vi "main.vi"() -> ()   [LabVIEW 2025]
uses:
  <userlib>/Nanonis Prog Interface V5/Nanonis Prog Interface.lvlib
panel:
  out "FRC":sgl format="%#_3g"
  out "CCR":sgl
  in  "Ref_filepath":path=path "si111-cornerhole.npy" caption="filename"
  in  "Final Overvew Details":T1={"Size (m)"={"Width"=nan, "Height"=nan}, "Pixels"=0, "Scan Speed (m/s)"=nan}
  in  "Shaping Attempt 5":T2={"Tip Lift (m)"=-1.3e-09, "Lifting Bias (V)"=5.0, "# Iterations"=20} caption="Tip Lift 1" {"# Iterations" step=1; "Lifting Bias (V)" step=0.5 format="%#_5g"; "Tip Lift (m)" step=5e-11 format="%.2p"}
  in  "Shaping Attempt 4":T2={"Tip Lift (m)"=-1.3e-09, "Lifting Bias (V)"=5.0, "# Iterations"=20} caption="Tip Lift 1" {"# Iterations" step=1; "Lifting Bias (V)" step=0.5 format="%#_5g"; "Tip Lift (m)" step=5e-11 format="%.2p"}
  in  "Shaping Attempt 3":T2={"Tip Lift (m)"=-1.3e-09, "Lifting Bias (V)"=5.0, "# Iterations"=20} caption="Tip Lift 1" {"# Iterations" step=1; "Lifting Bias (V)" step=0.5 format="%#_5g"; "Tip Lift (m)" step=5e-11 format="%.2p"}
  in  "Shaping Attempt 2":T2={"Tip Lift (m)"=-1.3e-09, "Lifting Bias (V)"=5.0, "# Iterations"=20} caption="Tip Lift 1" {"# Iterations" step=1; "Lifting Bias (V)" step=0.5 format="%#_5g"; "Tip Lift (m)" step=5e-11 format="%.2p"}
  in  "Tip Shaping Position":cluster{"X (m)":sgl, "Y (m)":sgl} {"X (m)" format="%#_6p"; "Y (m)" format="%#_6p"}
  out "Vy vs. Scan #":picture
  out "Vx vs. Scan #":picture
  out "Next filename":path caption="filename"
  in  "Ref Info":cluster{"Scan Size (m)":sgl, "Pixels":i32}={"Scan Size (m)"=2e-08, "Pixels"=720} {"Scan Size (m)" format="%#_4p"}
  out "Time \nElapsed (s)":dbl format="%#.2f"
  out "Shaping\nAttempts":i32
  in  "Shaping Attempt 1":T2={"Tip Lift (m)"=-1.3e-09, "Lifting Bias (V)"=5.0, "# Iterations"=20} caption="Tip Lift 1" {"# Iterations" step=1; "Lifting Bias (V)" step=0.5 format="%#_5g"; "Tip Lift (m)" step=5e-11 format="%.2p"}
  out "Finished?":bool
  in  "Start":bool
  # "Auto Tip Shaper"
  # "Tip Shaping Controls"
  # "Drift Plots"
  # "Pre-checks"
  # "See readme at https://github.com/DS-Barker/stm-tip-classifier for instructions"
  # "Final Overview Settings"
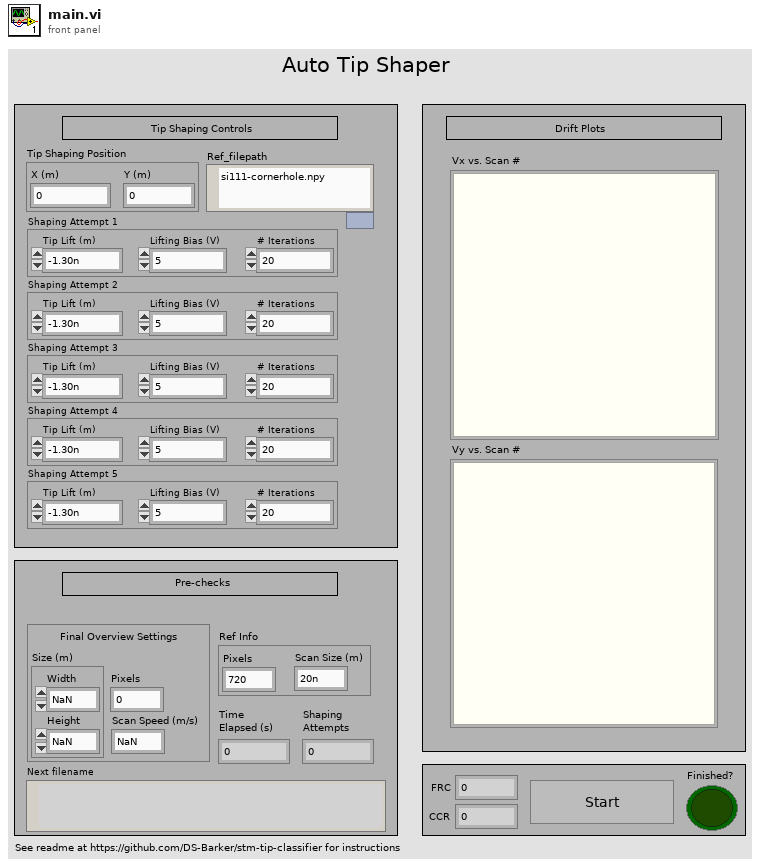
[diagram p1: front panel]
types:
  T1 = cluster{"Size (m)":cluster{"Width":sgl, "Height":sgl}, "Pixels":i32, "Scan Speed (m/s)":sgl}
  T2 = cluster{"Tip Lift (m)":dbl, "Lifting Bias (V)":dbl, "# Iterations":i32}
  T3 = cluster{cluster{"x":sgl, "y":sgl}[], cluster{"x":sgl, "y":sgl}[], cluster{"x":sgl, "y":sgl}[]}
  T4 = enum16{"Init", "Scanning", "Resolve Tip", "Shaping 1", "Shaping 2", "Shaping 3", "Shaping 4", "Shaping 5", "Move Away", "Quit"}
  T5 = cluster{"Application ref out":refnum<vi>, "error out":errorcluster, "Corner Coords":cluster{"Corner x":sgl, "Corner y":sgl}, "Tip Shaping Position":cluster{"Tip x (m)":sgl, "Tip y (m)":sgl}, "Session path":path, "Filenames":cluster{"Filename 1":path, "Filename 2":path}, "Downscale Info":cluster{"Scale factor":sgl, "Downscale ref/input":string}}
  T6 = cluster{"Scale factor":sgl, "Downscale ref/input":string}
  T7 = cluster{"Tip Lift 1 (m)":dbl, "Lift Time 1 (s)":dbl}
  T8 = cluster{"Bias Lift (V)":dbl, "Bias Settling Time (s)":dbl}
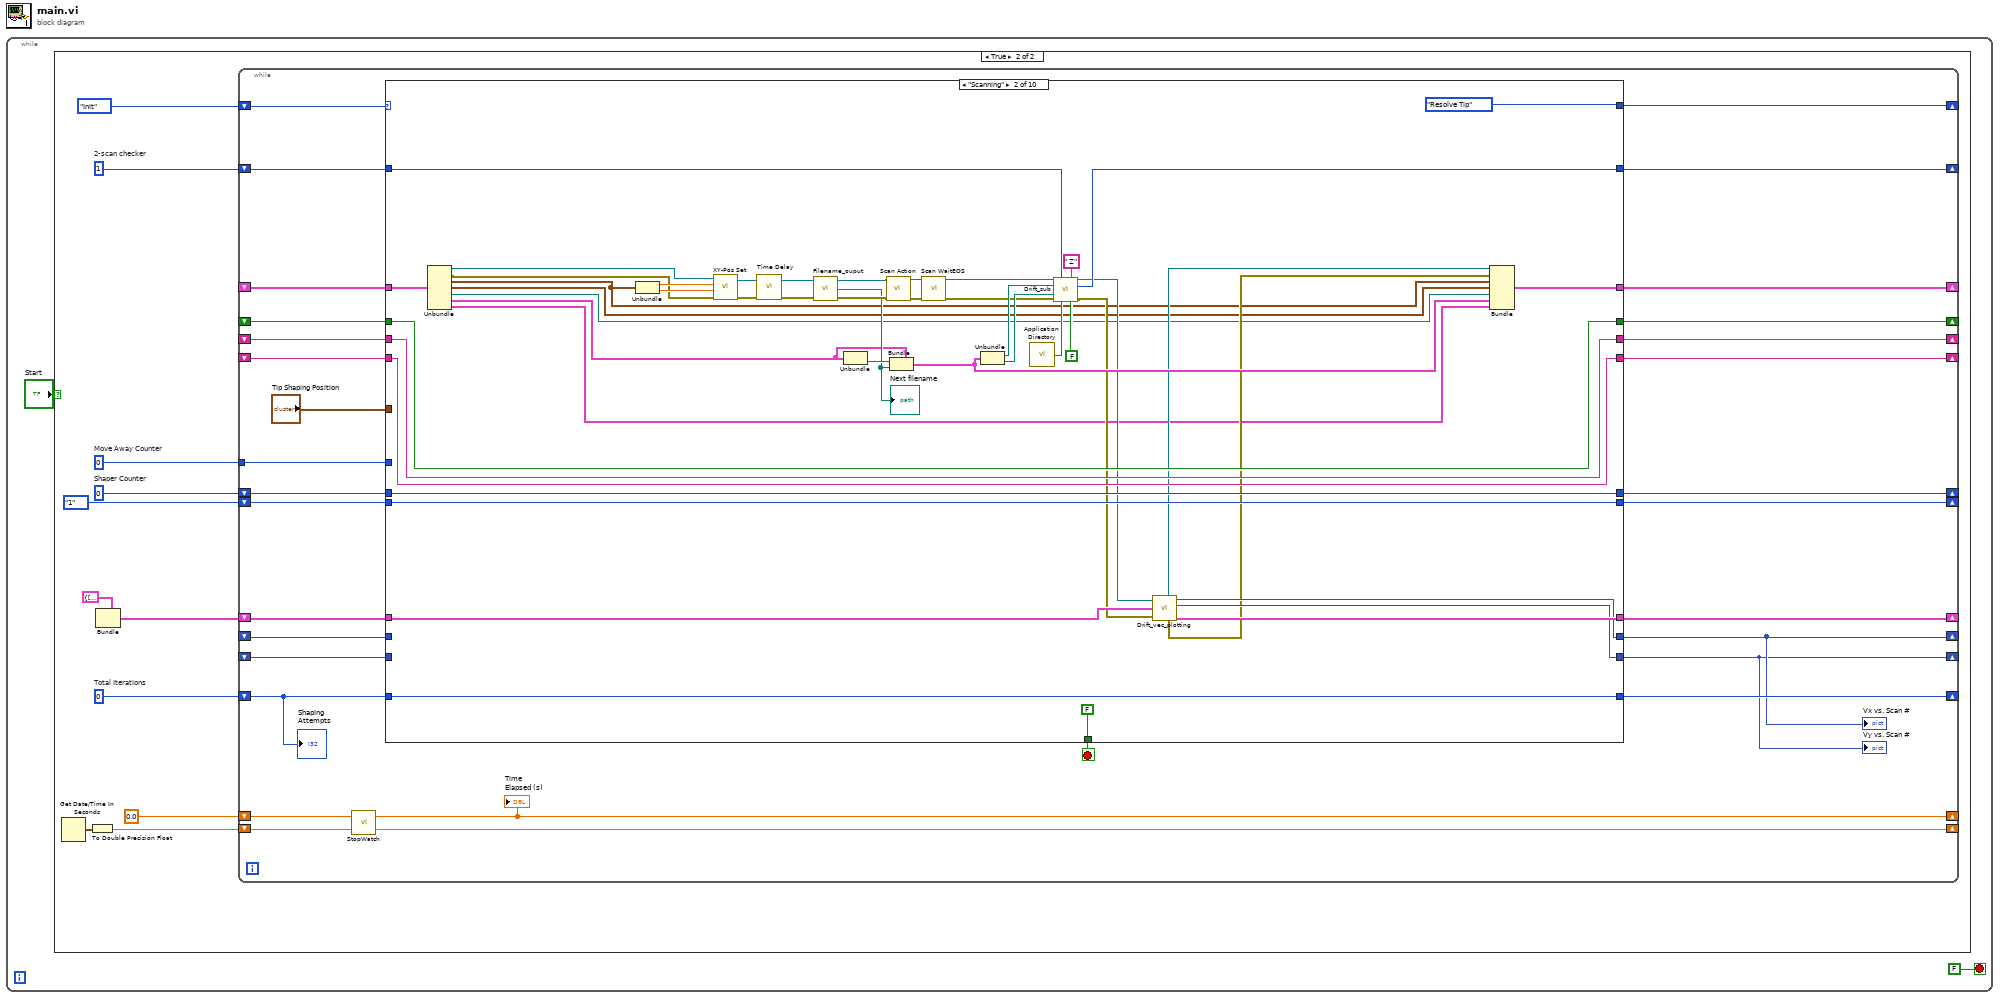
[diagram p0: block diagram]
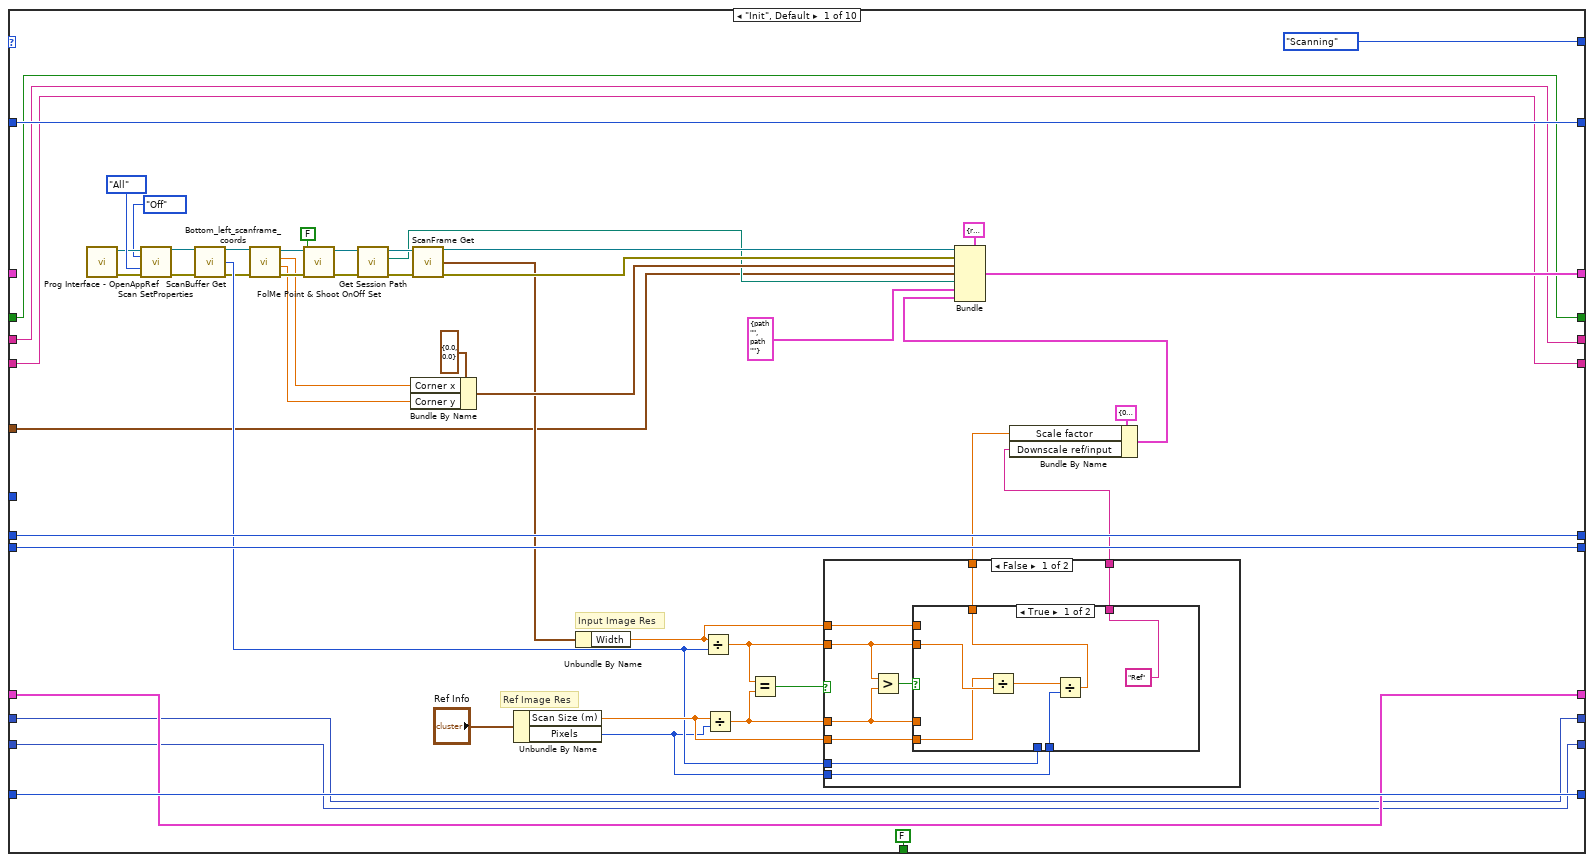
[diagram p3: hidden frame]
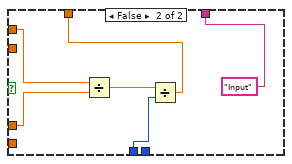
[diagram p4: hidden frame]
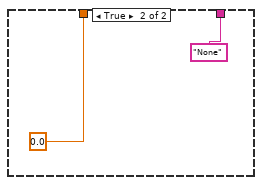
[diagram p5: hidden frame]
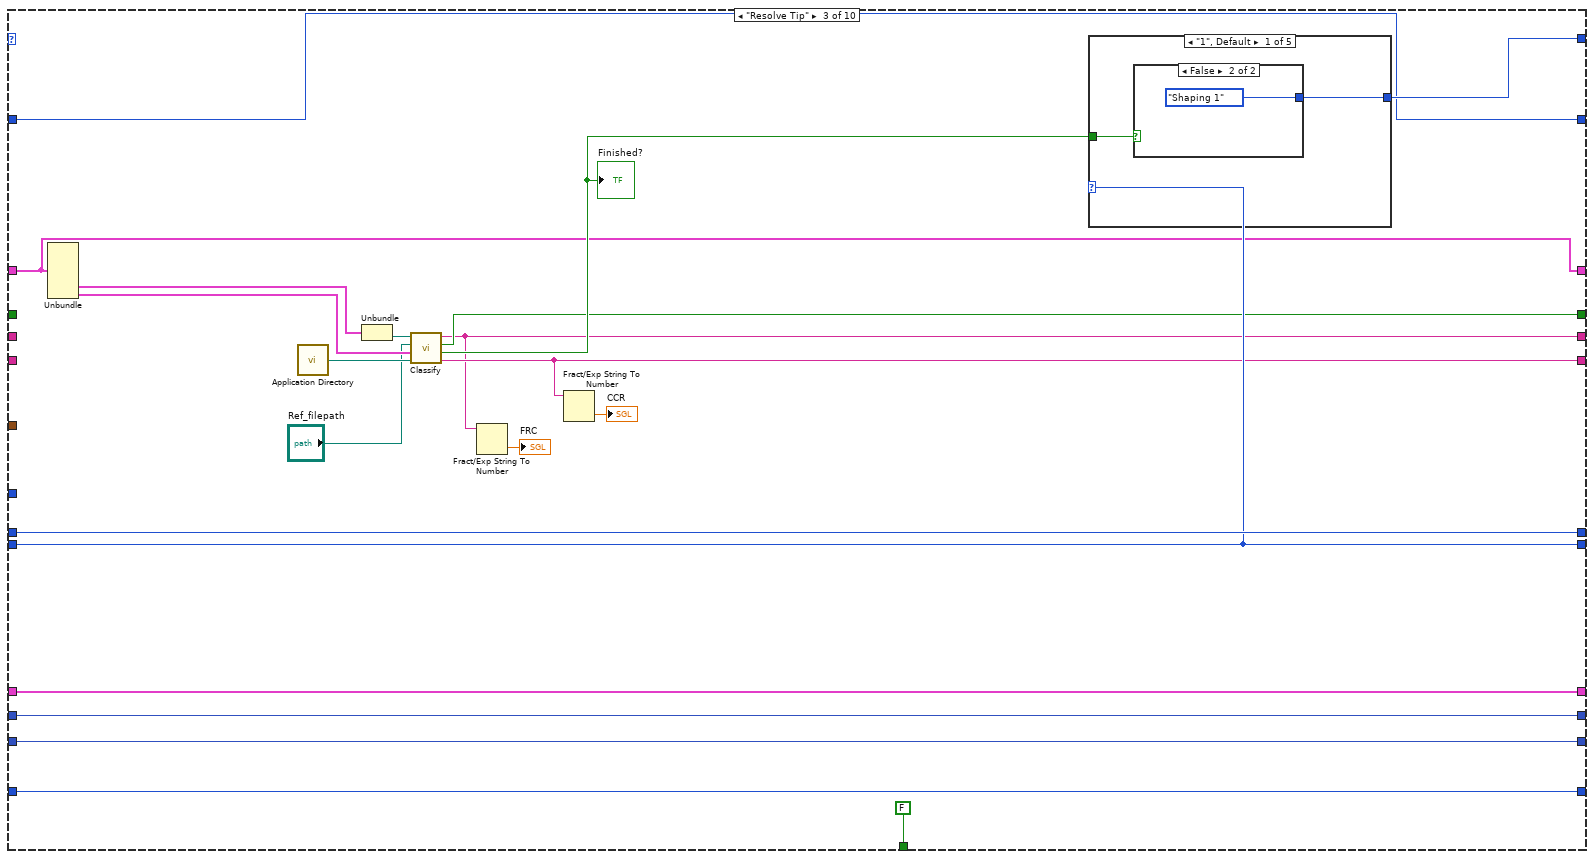
[diagram p6: hidden frame]
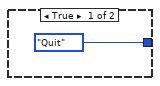
[diagram p7: hidden frame]
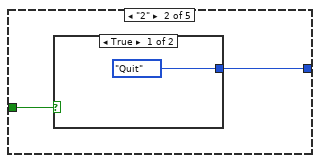
[diagram p8: hidden frame]
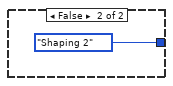
[diagram p9: hidden frame]
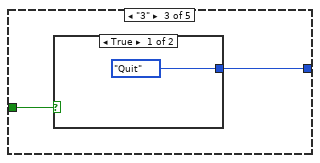
[diagram p10: hidden frame]
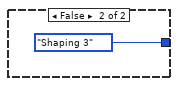
[diagram p11: hidden frame]
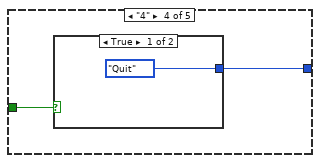
[diagram p12: hidden frame]
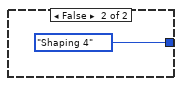
[diagram p13: hidden frame]
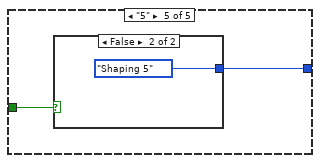
[diagram p14: hidden frame]
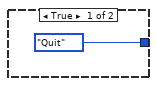
[diagram p15: hidden frame]
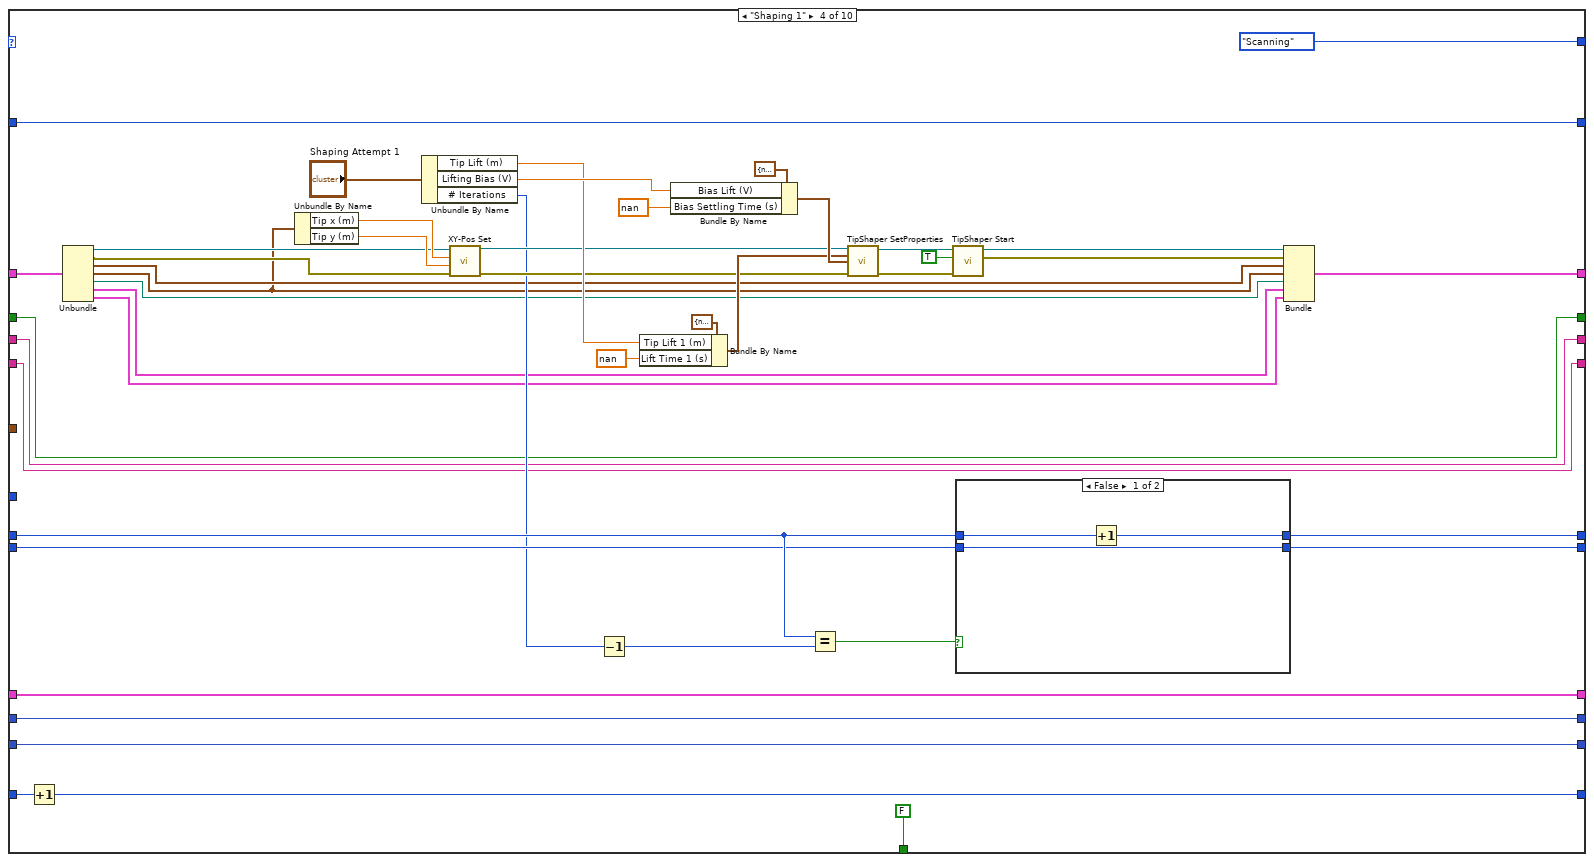
[diagram p16: hidden frame]
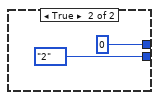
[diagram p17: hidden frame]
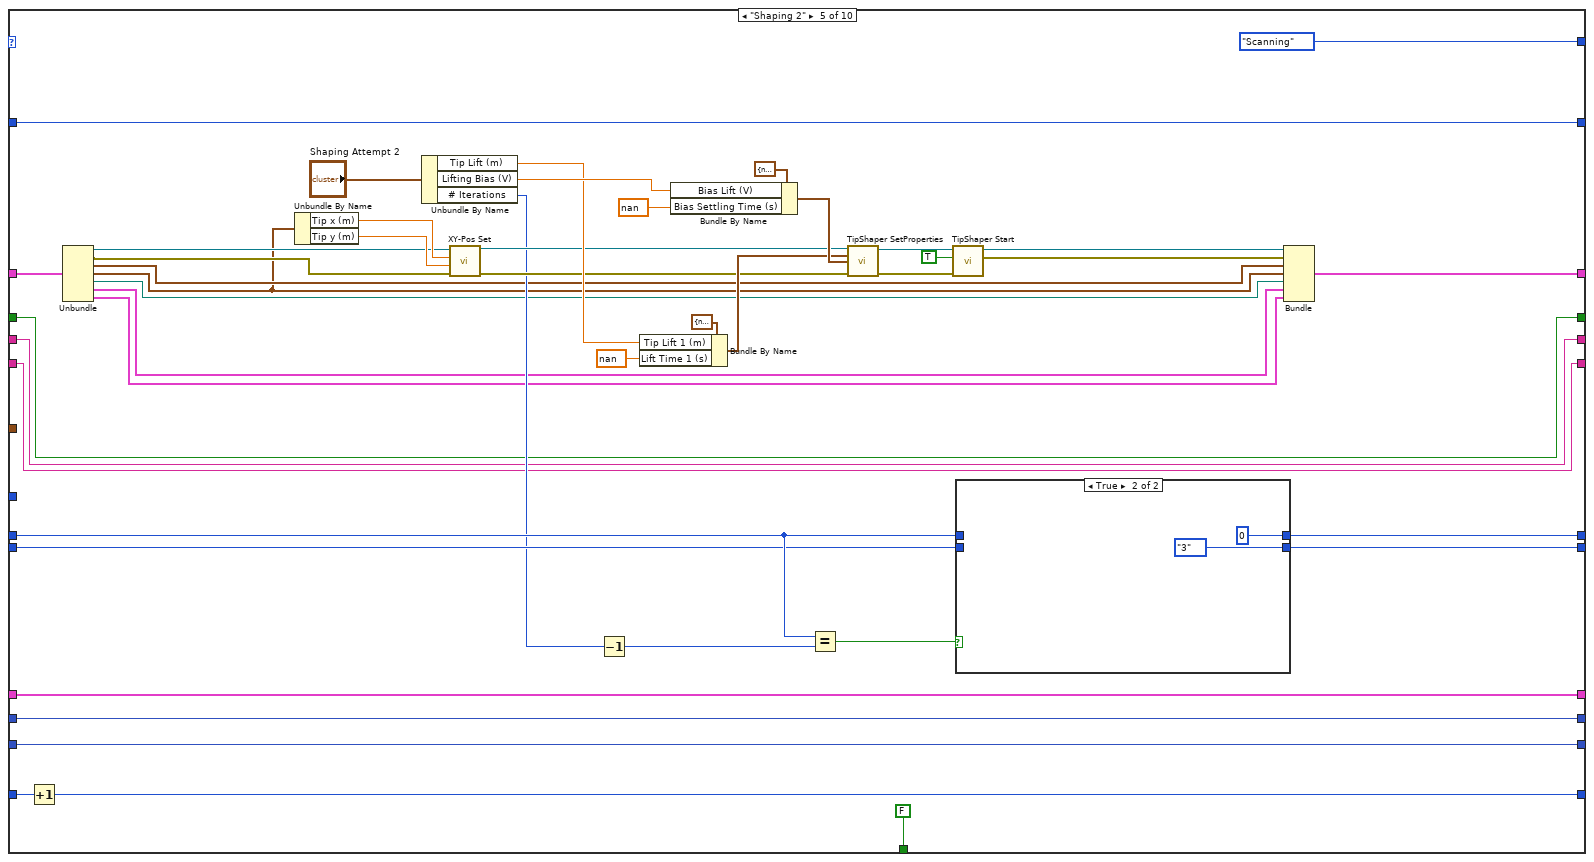
[diagram p18: hidden frame]
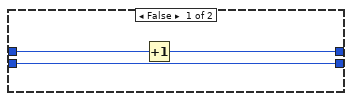
[diagram p19: hidden frame]
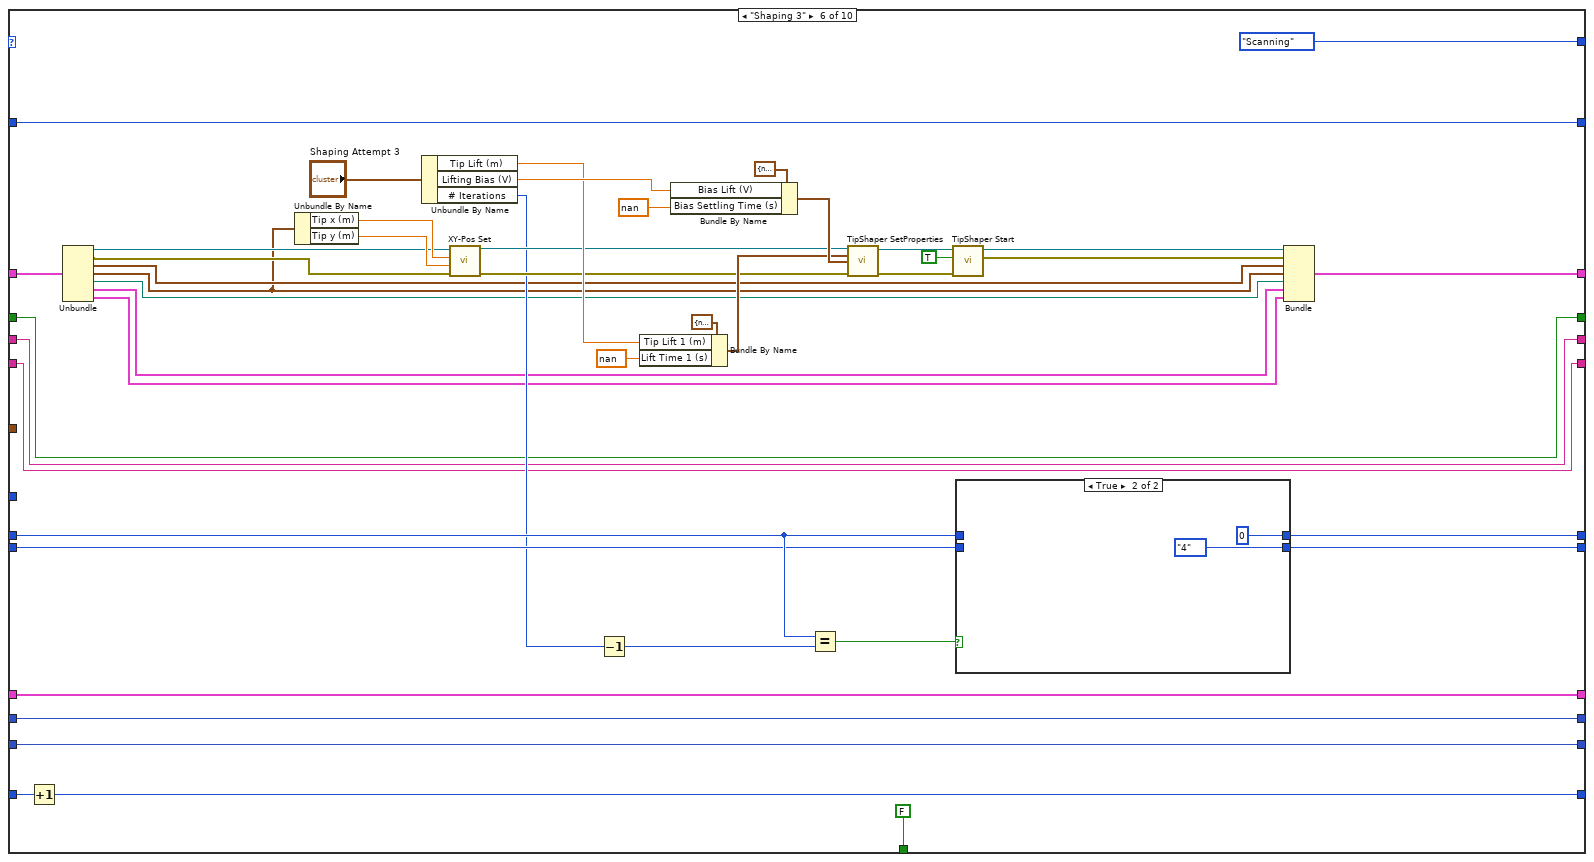
[diagram p20: hidden frame]
diagram:
  n1 = while {
    stop <- FALSE stop-if-true
    n2 = case shown="True" "Start" {
      frame False {
      }
      frame True {
        w5 = 1  # 2-scan checker
        w9 = 0  # Total Iterations
        w10 = 0  # Move Away Counter
        w12 = 0  # Shaper Counter
        n3 = Get Date/Time In Seconds() -> (seconds since 1Jan1904=w8:timestamp)
        n4 = To Double Precision Float(number=w8) -> (double precision float=w7:dbl)
        n5 = Bundle(cluster=T3 {[], [], []} ("output cluster")) -> (w4:T3)  [unwired: 3 in]
        n6 = while {
          shift-right: [w41] -> _
          shift-left: T4."Init" -> [w44]
          shift-right: [w43] -> _
          shift-left: _ -> [w42]
          shift-right: [w38] -> _
          shift-left: w12 -> [w39]
          shift-right: [w36] -> _
          shift-left: enum16{"1", "2", "3", "4", "5"}."1" -> [w37]
          tunnel: w10 -> [w35]
          shift-right: [w33] -> _
          shift-left: w9 -> [w34]
          shift-right: [w32] -> _
          shift-left: 0.0 ("Elapsed Time (Secs)") -> [w30]
          shift-right: [w31] -> _
          shift-left: w7 -> [w29]
          shift-right: [w27] -> _
          shift-left: w5 -> [w28]
          shift-right: [w25] -> _
          shift-left: w4 -> [w26]
          shift-right: [w24] -> _
          shift-left: _ -> [w22]
          shift-right: [w23] -> _
          shift-left: _ -> [w21]
          shift-right: [w18] -> _
          shift-left: _ -> [w15]
          shift-right: [w19] -> _
          shift-left: _ -> [w16]
          shift-right: [w20] -> _
          shift-left: _ -> [w17]
          stop <- w40 stop-if-true
          n7 = call "StopWatch.vi"("Global In (s)"=w29, "Elapsed In (s)"=w30) -> ("Global Out (s)"=w31:dbl, "Elapsed Time (Secs)"=w32:dbl)  [unwired: 1 in]
          "Time \nElapsed (s)" <- w32
          n8 = case shown="\"Scanning\"" w44 {
            selector: w44 -> [_ _ _ _ _ _ _ _ _ w533]
            tunnel: [w90 w159 w172 w232 w282 w332 w382 w432 w474 w507] -> w43
            tunnel: w42 -> [_ w126 w172 w213 w263 w313 w363 w414 w475 w513]
            tunnel: [T4."Scanning" T4."Resolve Tip" w184 T4."Scanning" T4."Scanning" T4."Scanning" T4."Scanning" w406 w467 w533] -> w41
            tunnel: [FALSE FALSE FALSE FALSE FALSE FALSE FALSE FALSE FALSE TRUE] -> w40
            tunnel: w39 -> [w85 w157 w183 w230 w280 w330 w380 w430 w473 w534]
            tunnel: [w85 w157 w183 w231 w281 w331 w381 w431 w473 w534] -> w38
            tunnel: w37 -> [w84 w156 w182 w226 w276 w326 w376 w427 w472 w531]
            tunnel: [w84 w156 w182 w228 w278 w328 w378 w428 w472 w531] -> w36
            tunnel: w35 -> [_ _ _ _ _ _ _ _ w471 _]
            tunnel: [w82 w154 w181 w221 w271 w321 w371 w422 w465 w532] -> w33
            tunnel: w34 -> [w82 w154 w181 w222 w272 w322 w372 w423 w465 w532]
            tunnel: w28 -> [w63 w146 w180 w220 w270 w320 w370 w421 w464 w530]
            tunnel: [w63 w145 w180 w220 w270 w320 w370 w421 w464 w530] -> w27
            tunnel: [w55 w132 w166 w215 w265 w315 w365 w416 w459 _] -> w19
            tunnel: [w54 w133 w168 w216 w266 w316 w366 w417 w460 _] -> w18
            tunnel: [w56 w131 w176 w214 w264 w314 w364 w415 w458 _] -> w20
            tunnel: [w59 w137 w175 w219 w269 w319 w369 w420 w463 w506] -> w25
            tunnel: [w58 w136 w174 w218 w268 w318 w368 w419 w462 w500] -> w24
            tunnel: [w57 w135 w173 w217 w267 w317 w367 w418 w461 w499] -> w23
            tunnel: w26 -> [w59 w134 w175 w219 w269 w319 w369 w420 w463 w506]
            tunnel: w22 -> [w58 _ w174 w218 w268 w318 w368 w419 w462 w500]
            tunnel: w21 -> [w57 _ w173 w217 w267 w317 w367 w418 w461 w499]
            tunnel: w17 -> [w56 w131 _ w214 w264 w314 w364 w415 w458 _]
            tunnel: w16 -> [w55 w132 _ w215 w265 w315 w365 w416 w459 _]
            tunnel: w15 -> [w54 w133 _ w216 w266 w316 w366 w417 w460 _]
            tunnel: "Tip Shaping Position" -> [w47 _ _ _ _ _ _ _ _ _]
            frame "Init", Default {
              # "Ref Image Res"
              # "Input Image Res"
              n9 = call <userlib>:"Prog Interface - OpenAppRef.vi"() -> ("Error out"=w93:errorcluster, "Application reference"=w94:refnum<vi>)  [unwired: 6 in]
              n10 = call <userlib>:"Scan SetProperties.vi"("Application ref in"=w94, "Continuous scan"=enum16{"No change", "On", "Off"}."Off", "Auto save"=enum16{"No change", "All", "Next", "Off"}."All", "Error in (no error)"=w93) -> ("Application ref out"=w76:refnum<vi>, "Error out"=w75:errorcluster)  [unwired: 10 in]
              n11 = call <userlib>:"ScanBuffer Get.vi"("Application ref in"=w76, "error in (no error)"=w75) -> ("Application ref out"=w53:refnum<vi>, "Pixels/line"=w62:i32, "error out"=w52:errorcluster)  [unwired: 9 in, 2 out]
              n12 = call "Bottom_left_scanframe_coords.vi"("error in"=w52, "Application ref in"=w53) -> ("error out"=w50:errorcluster, "Y_bl"=w48:sgl, "X_bl"=w49:sgl, "Application ref out"=w51:refnum<vi>)  [unwired: 2 in]
              n13 = call <userlib>:"FolMe Point & Shoot OnOff Set.vi"("error in (no error)"=w50, "Point & Shoot On/Off"=FALSE, "Application ref in"=w51) -> ("error out"=w80:errorcluster, "Application ref out"=w81:refnum<vi>)  [unwired: 7 in]
              n14 = call <userlib>:"Get Session Path.vi"("error in (no error)"=w80, "Application ref in"=w81) -> ("error out"=w78:errorcluster, "Session path"=w77:path, "Application ref out"=w79:refnum<vi>)  [unwired: 7 in]
              n15 = Bundle By Name(cluster=cluster{"Corner x":sgl, "Corner y":sgl} {"Corner x"=0.0, "Corner y"=0.0} ("Corner Coords"), "Corner x"=w49, "Corner y"=w48) -> (w87:cluster{"Corner x":sgl, "Corner y":sgl})
              n16 = call <userlib>:"ScanFrame Get.vi"("Application ref in"=w79, "error in (no error)"=w78) -> ("Application ref out"=w92:refnum<vi>, "Size (m)"=w74:cluster{"Width":sgl, "Height":sgl}, "error out"=w91:errorcluster)  [unwired: 9 in, 2 out]
              n17 = Unbundle By Name("Ref Info") -> ("Scan Size (m)"=w69:sgl, "Pixels"=w61:i32)
              n18 = Unbundle By Name(w74) -> ("Width"=w68:sgl)
              n19 = Divide(x=w68, y=w62) -> (x/y=w71:sgl)
              n20 = Divide(x=w69, y=w61) -> (x/y=w70:sgl)
              n21 = Equal?(x=w71, y=w70) -> (x = y?=w72:bool)
              n22 = case shown="False" w72 {
                tunnel: w71 -> [w103 _]
                tunnel: w70 -> [w102 _]
                tunnel: w69 -> [w100 _]
                tunnel: w68 -> [w101 _]
                tunnel: [w99 "None"] -> w66
                tunnel: w62 -> [w98 _]
                tunnel: w61 -> [w97 _]
                tunnel: [w96 sgl 0.0] -> w60
                frame False {
                  n23 = Greater?(x=w103, y=w102) -> (0:w104:bool)
                  n24 = case shown="True" w104 {
                    tunnel: w103 -> [w110 _]
                    tunnel: w102 -> [_ w115]
                    tunnel: w101 -> [_ w116]
                    tunnel: w100 -> [w109 _]
                    tunnel: ["Ref" "Input"] -> w99
                    tunnel: w98 -> [_ w112]
                    tunnel: w97 -> [w106 _]
                    tunnel: [w105 w111] -> w96
                    frame True {
                      n25 = Divide(x=w109, y=w110) -> (x/y=w107:sgl)
                      n26 = Divide(x=w107, y=w106) -> (x/y=w105:sgl)
                    }
                    frame False {
                      n27 = Divide(x=w116, y=w115) -> (x/y=w113:sgl)
                      n28 = Divide(x=w113, y=w112) -> (x/y=w111:sgl)
                    }
                  }
                }
                frame True {
                }
              }
              n29 = Bundle By Name(cluster=T6 {"Scale factor"=0.0, "Downscale ref/input"=""} ("Downscale Info"), "Scale factor"=w60, "Downscale ref/input"=w66) -> (w65:T6)
              n30 = Bundle(cluster=T5 {"Application ref out"=refnum, "error out"={"status"=FALSE, "code"=0, "source"=""}, "Corner Coords"={"Corner x"=0.0, "Corner y"=0.0}, "Tip Shaping Position"={"Tip x (m)"=0.0, "Tip y (m)"=0.0}, "Session path"=path "", "Filenames"={"Filename 1"=path "", "Filename 2"=path ""}, "Downscale Info"={"Scale factor"=0.0, "Downscale ref/input"=""}}, "Application ref out"=w92, "error out"=w91, "Corner Coords"=w87, "Tip Shaping Position"=w47, "Session path"=w77, "Filenames"=cluster{"Filename 1":path, "Filename 2":path} {"Filename 1"=path "", "Filename 2"=path ""}, "Downscale Info"=w65) -> (w90:T5)
            }
            frame "Scanning" {
              n31 = Unbundle(w126) -> ("Application ref out"=w125:refnum<vi>, "error out"=w124:errorcluster, "Corner Coords"=w123:cluster{"Corner x":sgl, "Corner y":sgl}, "Tip Shaping Position"=w122:cluster{"Tip x (m)":sgl, "Tip y (m)":sgl}, "Session path"=w121:path, "Filenames"=w120:cluster{"Filename 1":path, "Filename 2":path}, "Downscale Info"=w119:T6)
              n32 = Unbundle(w123) -> ("Corner x"=w164:sgl, "Corner y"=w163:sgl)
              n33 = call <userlib>:"XY-Pos Set.vi"("error in (no error)"=w124, "Y (m)"=w163, "X (m)"=w164, "Application ref in"=w125) -> ("error out"=w162:errorcluster, "Application ref out"=w151:refnum<vi>)  [unwired: 4 in]
              n34 = call "Time Delay"("error in (no error)"=w162) -> ("error out"=w150:errorcluster)  [unwired: 10 in]
              n35 = call "Filename_ouput.vi"("Error in (no error)"=w150, "Application ref in"=w151) -> ("error out"=w152:errorcluster, "Next filename"=w148:path, "Application ref out"=w153:refnum<vi>)  [unwired: 1 in]
              "Next filename" <- w148
              n36 = Unbundle(w120) -> ("Filename 2"=w149:path)  [unwired: 1 out]
              n37 = call <userlib>:"Scan Action.vi"("error in (no error)"=w152, "Application ref in"=w153) -> ("error out"=w161:errorcluster, "Application ref out"=w160:refnum<vi>)  [unwired: 7 in]
              n38 = Bundle(cluster=w120, "Filename 1"=w149, "Filename 2"=w148) -> (w147:cluster{"Filename 1":path, "Filename 2":path})
              n39 = call <userlib>:"Scan WaitEOS.vi"("error in (no error)"=w161, "Application ref in"=w160) -> ("error out"=w141:errorcluster, "Application ref out"=w144:refnum<vi>)  [unwired: 5 in, 2 out]
              n40 = Unbundle(w147) -> ("Filename 1"=w143:path, "Filename 2"=w142:path)
              n41 = call <vilib>:"Application Directory.vi"() -> ("Application Directory"=w139:path)
              n42 = call "Drift_sub.vi"("Application ref in"=w144, "2-scan checker in"=w146, "Image Channel"=" Z", "Filename_1"=w143, "Filename_2"=w142, "error in"=w141, "Python Directory Path"=w139, "Z-Compensation?"=FALSE) -> ("Application ref out"=w130:refnum<vi>, "2-scan checker out"=w145:i32, "error out"=w128:errorcluster)  [unwired: 5 in]
              n43 = call "Drift_vec_plotting.vi"("Application ref in"=w130, "Plotting Data In"=w134, "error in"=w128) -> ("Application ref out"=w129:refnum<vi>, "Vx vs. Scan #"=w136:picture, "Vy vs. Scan #"=w135:picture, "error out"=w127:errorcluster, "Plotting Data Out"=w137:T3)  [unwired: 2 in, 1 out]
              n44 = Bundle("Application ref out"=w129, "error out"=w127, "Corner Coords"=w123, "Tip Shaping Position"=w122, "Session path"=w121, "Filenames"=w147, "Downscale Info"=w119) -> (w159:T5)  [unwired: 1 in]
            }
            frame "Resolve Tip" {
              n45 = Unbundle(w172) -> ("Filenames"=w171:cluster{"Filename 1":path, "Filename 2":path}, "Downscale Info"=w170:T6)  [unwired: 5 out]
              n46 = call <vilib>:"Application Directory.vi"() -> ("Application Directory"=w179:path)
              n47 = Unbundle(w171) -> ("Filename 2"=w177:path)  [unwired: 1 out]
              n48 = call "Classify.vi"("Python Directory Path"=w179, "input cluster"=w170, "Ref_filepath"="Ref_filepath", "Filename_1"=w177) -> ("CCR"=w168:string, "Good Image"=w178:bool, "Tip Change?"=w176:bool, "FRC"=w166:string)
              "Finished?" <- w178
              n49 = Fract/Exp String To Number(string=w166) -> (number=→"FRC":dbl)  [unwired: 3 in, 1 out]
              n50 = Fract/Exp String To Number(string=w168) -> (number=→"CCR":dbl)  [unwired: 3 in, 1 out]
              n51 = case shown="\"1\", Default" w182 {
                tunnel: w178 -> [w187 w191 w195 w199 w203]
                tunnel: [w186 w190 w194 w198 w202] -> w184
                frame "1", Default {
                  n52 = case shown="False" w187 {
                    tunnel: [T4."Quit" T4."Shaping 1"] -> w186
                    frame True {
                    }
                    frame False {
                    }
                  }
                }
                frame "2" {
                  n53 = case shown="True" w191 {
                    tunnel: [T4."Quit" T4."Shaping 2"] -> w190
                    frame True {
                    }
                    frame False {
                    }
                  }
                }
                frame "3" {
                  n54 = case shown="True" w195 {
                    tunnel: [T4."Quit" T4."Shaping 3"] -> w194
                    frame True {
                    }
                    frame False {
                    }
                  }
                }
                frame "4" {
                  n55 = case shown="True" w199 {
                    tunnel: [T4."Quit" T4."Shaping 4"] -> w198
                    frame True {
                    }
                    frame False {
                    }
                  }
                }
                frame "5" {
                  n56 = case shown="False" w203 {
                    tunnel: [T4."Quit" T4."Shaping 5"] -> w202
                    frame True {
                    }
                    frame False {
                    }
                  }
                }
              }
            }
            frame "Shaping 1" {
              n57 = Increment(x=w222) -> (x+1=w221:i32)
              n58 = Unbundle(w213) -> ("Application ref out"=w212:refnum<vi>, "error out"=w211:errorcluster, "Corner Coords"=w210:cluster{"Corner x":sgl, "Corner y":sgl}, "Tip Shaping Position"=w209:cluster{"Tip x (m)":sgl, "Tip y (m)":sgl}, "Session path"=w208:path, "Filenames"=w207:cluster{"Filename 1":path, "Filename 2":path}, "Downscale Info"=w206:T6)
              n59 = Unbundle By Name(w209) -> ("Tip x (m)"=w238:sgl, "Tip y (m)"=w237:sgl)
              n60 = Unbundle By Name("Shaping Attempt 1") -> ("Tip Lift (m)"=w244:dbl, "Lifting Bias (V)"=w247:dbl, "# Iterations"=w223:i32)
              n61 = call <userlib>:"XY-Pos Set.vi"("error in (no error)"=w211, "Y (m)"=w237, "X (m)"=w238, "Application ref in"=w212) -> ("error out"=w235:errorcluster, "Application ref out"=w236:refnum<vi>)  [unwired: 4 in]
              n62 = Decrement(x=w223) -> (x-1=w224:i32)
              n63 = Bundle By Name(cluster=T7 {"Tip Lift 1 (m)"=nan, "Lift Time 1 (s)"=nan} ("Tip Lift 1"), "Tip Lift 1 (m)"=w244, "Lift Time 1 (s)"=nan) -> (w242:T7)
              n64 = Bundle By Name(cluster=T8 {"Bias Lift (V)"=nan, "Bias Settling Time (s)"=nan} ("Bias Lift"), "Bias Lift (V)"=w247, "Bias Settling Time (s)"=nan) -> (w246:T8)
              n65 = Equal?(x=w230, y=w224) -> (x = y?=w229:bool)
              n66 = call <userlib>:"TipShaper SetProperties.vi"("Application ref in"=w236, "Tip Lift 1"=w242, "Bias Lift"=w246, "Error in (no error)"=w235) -> ("Application ref out"=w241:refnum<vi>, "Error out"=w240:errorcluster)  [unwired: 10 in]
              n67 = call <userlib>:"TipShaper Start.vi"("error in (no error)"=w240, "Wait until finished? (F)"=TRUE, "Application ref in"=w241) -> ("error out"=w233:errorcluster, "Application ref out"=w234:refnum<vi>)  [unwired: 6 in]
              n68 = case shown="False" w229 {
                tunnel: w230 -> [w253 _]
                tunnel: [w252 0] -> w231
                tunnel: [w251 enum16{"1", "2", "3", "4", "5"}."2"] -> w228
                tunnel: w226 -> [w251 _]
                frame False {
                  n69 = Increment(x=w253) -> (x+1=w252:i32)
                }
                frame True {
                }
              }
              n70 = Bundle("Application ref out"=w234, "error out"=w233, "Corner Coords"=w210, "Tip Shaping Position"=w209, "Session path"=w208, "Filenames"=w207, "Downscale Info"=w206) -> (w232:T5)  [unwired: 1 in]
            }
            frame "Shaping 2" {
              n71 = Increment(x=w272) -> (x+1=w271:i32)
              n72 = Unbundle(w263) -> ("Application ref out"=w262:refnum<vi>, "error out"=w261:errorcluster, "Corner Coords"=w260:cluster{"Corner x":sgl, "Corner y":sgl}, "Tip Shaping Position"=w259:cluster{"Tip x (m)":sgl, "Tip y (m)":sgl}, "Session path"=w258:path, "Filenames"=w257:cluster{"Filename 1":path, "Filename 2":path}, "Downscale Info"=w256:T6)
              n73 = Unbundle By Name(w259) -> ("Tip x (m)"=w288:sgl, "Tip y (m)"=w287:sgl)
              n74 = Unbundle By Name("Shaping Attempt 2") -> ("Tip Lift (m)"=w294:dbl, "Lifting Bias (V)"=w297:dbl, "# Iterations"=w273:i32)
              n75 = call <userlib>:"XY-Pos Set.vi"("error in (no error)"=w261, "Y (m)"=w287, "X (m)"=w288, "Application ref in"=w262) -> ("error out"=w285:errorcluster, "Application ref out"=w286:refnum<vi>)  [unwired: 4 in]
              n76 = Decrement(x=w273) -> (x-1=w274:i32)
              n77 = Bundle By Name(cluster=T7 {"Tip Lift 1 (m)"=nan, "Lift Time 1 (s)"=nan} ("Tip Lift 1"), "Tip Lift 1 (m)"=w294, "Lift Time 1 (s)"=nan) -> (w292:T7)
              n78 = Bundle By Name(cluster=T8 {"Bias Lift (V)"=nan, "Bias Settling Time (s)"=nan} ("Bias Lift"), "Bias Lift (V)"=w297, "Bias Settling Time (s)"=nan) -> (w296:T8)
              n79 = Equal?(x=w280, y=w274) -> (x = y?=w279:bool)
              n80 = call <userlib>:"TipShaper SetProperties.vi"("Application ref in"=w286, "Tip Lift 1"=w292, "Bias Lift"=w296, "Error in (no error)"=w285) -> ("Application ref out"=w291:refnum<vi>, "Error out"=w290:errorcluster)  [unwired: 10 in]
              n81 = call <userlib>:"TipShaper Start.vi"("error in (no error)"=w290, "Wait until finished? (F)"=TRUE, "Application ref in"=w291) -> ("error out"=w283:errorcluster, "Application ref out"=w284:refnum<vi>)  [unwired: 6 in]
              n82 = case shown="True" w279 {
                tunnel: w280 -> [w303 _]
                tunnel: [w302 0] -> w281
                tunnel: [w301 enum16{"1", "2", "3", "4", "5"}."3"] -> w278
                tunnel: w276 -> [w301 _]
                frame False {
                  n83 = Increment(x=w303) -> (x+1=w302:i32)
                }
                frame True {
                }
              }
              n84 = Bundle("Application ref out"=w284, "error out"=w283, "Corner Coords"=w260, "Tip Shaping Position"=w259, "Session path"=w258, "Filenames"=w257, "Downscale Info"=w256) -> (w282:T5)  [unwired: 1 in]
            }
            frame "Shaping 3" {
              n85 = Increment(x=w322) -> (x+1=w321:i32)
              n86 = Unbundle(w313) -> ("Application ref out"=w312:refnum<vi>, "error out"=w311:errorcluster, "Corner Coords"=w310:cluster{"Corner x":sgl, "Corner y":sgl}, "Tip Shaping Position"=w309:cluster{"Tip x (m)":sgl, "Tip y (m)":sgl}, "Session path"=w308:path, "Filenames"=w307:cluster{"Filename 1":path, "Filename 2":path}, "Downscale Info"=w306:T6)
              n87 = Unbundle By Name(w309) -> ("Tip x (m)"=w338:sgl, "Tip y (m)"=w337:sgl)
              n88 = Unbundle By Name("Shaping Attempt 3") -> ("Tip Lift (m)"=w344:dbl, "Lifting Bias (V)"=w347:dbl, "# Iterations"=w323:i32)
              n89 = call <userlib>:"XY-Pos Set.vi"("error in (no error)"=w311, "Y (m)"=w337, "X (m)"=w338, "Application ref in"=w312) -> ("error out"=w335:errorcluster, "Application ref out"=w336:refnum<vi>)  [unwired: 4 in]
              n90 = Decrement(x=w323) -> (x-1=w324:i32)
              n91 = Bundle By Name(cluster=T7 {"Tip Lift 1 (m)"=nan, "Lift Time 1 (s)"=nan} ("Tip Lift 1"), "Tip Lift 1 (m)"=w344, "Lift Time 1 (s)"=nan) -> (w342:T7)
              n92 = Bundle By Name(cluster=T8 {"Bias Lift (V)"=nan, "Bias Settling Time (s)"=nan} ("Bias Lift"), "Bias Lift (V)"=w347, "Bias Settling Time (s)"=nan) -> (w346:T8)
              n93 = Equal?(x=w330, y=w324) -> (x = y?=w329:bool)
              n94 = call <userlib>:"TipShaper SetProperties.vi"("Application ref in"=w336, "Tip Lift 1"=w342, "Bias Lift"=w346, "Error in (no error)"=w335) -> ("Application ref out"=w341:refnum<vi>, "Error out"=w340:errorcluster)  [unwired: 10 in]
              n95 = call <userlib>:"TipShaper Start.vi"("error in (no error)"=w340, "Wait until finished? (F)"=TRUE, "Application ref in"=w341) -> ("error out"=w333:errorcluster, "Application ref out"=w334:refnum<vi>)  [unwired: 6 in]
              n96 = case shown="True" w329 {
                tunnel: w330 -> [w353 _]
                tunnel: [w352 0] -> w331
                tunnel: [w351 enum16{"1", "2", "3", "4", "5"}."4"] -> w328
                tunnel: w326 -> [w351 _]
                frame False {
                  n97 = Increment(x=w353) -> (x+1=w352:i32)
                }
                frame True {
                }
              }
              n98 = Bundle("Application ref out"=w334, "error out"=w333, "Corner Coords"=w310, "Tip Shaping Position"=w309, "Session path"=w308, "Filenames"=w307, "Downscale Info"=w306) -> (w332:T5)  [unwired: 1 in]
            }
            frame "Shaping 4" {
              n99 = Increment(x=w372) -> (x+1=w371:i32)
              n100 = Unbundle(w363) -> ("Application ref out"=w362:refnum<vi>, "error out"=w361:errorcluster, "Corner Coords"=w360:cluster{"Corner x":sgl, "Corner y":sgl}, "Tip Shaping Position"=w359:cluster{"Tip x (m)":sgl, "Tip y (m)":sgl}, "Session path"=w358:path, "Filenames"=w357:cluster{"Filename 1":path, "Filename 2":path}, "Downscale Info"=w356:T6)
              n101 = Unbundle By Name(w359) -> ("Tip x (m)"=w388:sgl, "Tip y (m)"=w387:sgl)
              n102 = Unbundle By Name("Shaping Attempt 4") -> ("Tip Lift (m)"=w394:dbl, "Lifting Bias (V)"=w397:dbl, "# Iterations"=w373:i32)
              n103 = call <userlib>:"XY-Pos Set.vi"("error in (no error)"=w361, "Y (m)"=w387, "X (m)"=w388, "Application ref in"=w362) -> ("error out"=w385:errorcluster, "Application ref out"=w386:refnum<vi>)  [unwired: 4 in]
              n104 = Decrement(x=w373) -> (x-1=w374:i32)
              n105 = Bundle By Name(cluster=T7 {"Tip Lift 1 (m)"=nan, "Lift Time 1 (s)"=nan} ("Tip Lift 1"), "Tip Lift 1 (m)"=w394, "Lift Time 1 (s)"=nan) -> (w392:T7)
              n106 = Bundle By Name(cluster=T8 {"Bias Lift (V)"=nan, "Bias Settling Time (s)"=nan} ("Bias Lift"), "Bias Lift (V)"=w397, "Bias Settling Time (s)"=nan) -> (w396:T8)
              n107 = Equal?(x=w380, y=w374) -> (x = y?=w379:bool)
              n108 = call <userlib>:"TipShaper SetProperties.vi"("Application ref in"=w386, "Tip Lift 1"=w392, "Bias Lift"=w396, "Error in (no error)"=w385) -> ("Application ref out"=w391:refnum<vi>, "Error out"=w390:errorcluster)  [unwired: 10 in]
              n109 = call <userlib>:"TipShaper Start.vi"("error in (no error)"=w390, "Wait until finished? (F)"=TRUE, "Application ref in"=w391) -> ("error out"=w383:errorcluster, "Application ref out"=w384:refnum<vi>)  [unwired: 6 in]
              n110 = case shown="True" w379 {
                tunnel: w380 -> [w403 _]
                tunnel: [w402 0] -> w381
                tunnel: [w401 enum16{"1", "2", "3", "4", "5"}."5"] -> w378
                tunnel: w376 -> [w401 _]
                frame False {
                  n111 = Increment(x=w403) -> (x+1=w402:i32)
                }
                frame True {
                }
              }
              n112 = Bundle("Application ref out"=w384, "error out"=w383, "Corner Coords"=w360, "Tip Shaping Position"=w359, "Session path"=w358, "Filenames"=w357, "Downscale Info"=w356) -> (w382:T5)  [unwired: 1 in]
            }
            frame "Shaping 5" {
              n113 = Increment(x=w423) -> (x+1=w422:i32)
              n114 = Unbundle(w414) -> ("Application ref out"=w413:refnum<vi>, "error out"=w412:errorcluster, "Corner Coords"=w411:cluster{"Corner x":sgl, "Corner y":sgl}, "Tip Shaping Position"=w410:cluster{"Tip x (m)":sgl, "Tip y (m)":sgl}, "Session path"=w409:path, "Filenames"=w408:cluster{"Filename 1":path, "Filename 2":path}, "Downscale Info"=w407:T6)
              n115 = Unbundle By Name(w410) -> ("Tip x (m)"=w438:sgl, "Tip y (m)"=w437:sgl)
              n116 = Unbundle By Name("Shaping Attempt 5") -> ("Tip Lift (m)"=w444:dbl, "Lifting Bias (V)"=w447:dbl, "# Iterations"=w424:i32)
              n117 = call <userlib>:"XY-Pos Set.vi"("error in (no error)"=w412, "Y (m)"=w437, "X (m)"=w438, "Application ref in"=w413) -> ("error out"=w435:errorcluster, "Application ref out"=w436:refnum<vi>)  [unwired: 4 in]
              n118 = Decrement(x=w424) -> (x-1=w425:i32)
              n119 = Bundle By Name(cluster=T7 {"Tip Lift 1 (m)"=nan, "Lift Time 1 (s)"=nan} ("Tip Lift 1"), "Tip Lift 1 (m)"=w444, "Lift Time 1 (s)"=nan) -> (w442:T7)
              n120 = Bundle By Name(cluster=T8 {"Bias Lift (V)"=nan, "Bias Settling Time (s)"=nan} ("Bias Lift"), "Bias Lift (V)"=w447, "Bias Settling Time (s)"=nan) -> (w446:T8)
              n121 = Equal?(x=w430, y=w425) -> (x = y?=w429:bool)
              n122 = call <userlib>:"TipShaper SetProperties.vi"("Application ref in"=w436, "Tip Lift 1"=w442, "Bias Lift"=w446, "Error in (no error)"=w435) -> ("Application ref out"=w441:refnum<vi>, "Error out"=w440:errorcluster)  [unwired: 10 in]
              n123 = call <userlib>:"TipShaper Start.vi"("error in (no error)"=w440, "Wait until finished? (F)"=TRUE, "Application ref in"=w441) -> ("error out"=w433:errorcluster, "Application ref out"=w434:refnum<vi>)  [unwired: 6 in]
              n124 = case shown="True" w429 {
                tunnel: w430 -> [w454 _]
                tunnel: [w453 0] -> w431
                tunnel: [w452 enum16{"1", "2", "3", "4", "5"}."1"] -> w428
                tunnel: w427 -> [w452 _]
                tunnel: [T4."Scanning" T4."Quit"] -> w406
                frame False {
                  n125 = Increment(x=w454) -> (x+1=w453:i32)
                }
                frame True {
                }
              }
              n126 = Bundle("Application ref out"=w434, "error out"=w433, "Corner Coords"=w411, "Tip Shaping Position"=w410, "Session path"=w409, "Filenames"=w408, "Downscale Info"=w407) -> (w432:T5)  [unwired: 1 in]
            }
            frame "Move Away" {
              n127 = Increment(x=w471) -> (x+1=w470:i32)
              n128 = Equal?(x=3, y=w470) -> (x = y?=w469:bool)
              n129 = case shown="True" w469 {
                tunnel: w475 -> [w477 w485]
                tunnel: [w477 w487] -> w474
                tunnel: [T4."Quit" T4."Scanning"] -> w467
                frame True {
                }
                frame False {
                  # "Moving away if no good tip by final shaping attempt"
                  n130 = Unbundle(w485) -> ("Application ref out"=w484:refnum<vi>, "error out"=w483:errorcluster, "Corner Coords"=w482:cluster{"Corner x":sgl, "Corner y":sgl}, "Tip Shaping Position"=w481:cluster{"Tip x (m)":sgl, "Tip y (m)":sgl}, "Session path"=w480:path, "Filenames"=w479:cluster{"Filename 1":path, "Filename 2":path}, "Downscale Info"=w478:T6)
                  n131 = call <userlib>:"Withdraw.vi"("Wait until finished? (default=False)"=TRUE, "Error in (no error)"=w483, "Application ref in"=w484) -> ("Error out"=w494:errorcluster, "Application ref out"=w495:refnum<vi>)  [unwired: 7 in]
                  n132 = call <userlib>:"Motor Start Move.vi"("Wait until finished? (F)"=TRUE, "Error in (no error)"=w494, "Number of steps"=u16 10, "Direction"=enum16{"X +", "X -", "Y +", "Y -", "Z +", "Z -"}."X -", "Application ref in"=w495) -> ("Error out"=w492:errorcluster, "Application ref out"=w491:refnum<vi>)  [unwired: 4 in]
                  n133 = call <userlib>:"Ctrl-on_off Set.vi"("error in (no error)"=w492, "Z Controller ON/OFF"=TRUE, "Application ref in"=w491) -> ("error out"=w488:errorcluster, "Application ref out"=w489:refnum<vi>)  [unwired: 7 in]
                  n134 = Bundle("Application ref out"=w489, "error out"=w488, "Corner Coords"=w482, "Tip Shaping Position"=w481, "Session path"=w480, "Filenames"=w479, "Downscale Info"=w478) -> (w487:T5)  [unwired: 1 in]
                }
              }
            }
            frame "Quit" {
              n135 = Unbundle(w513) -> ("Application ref out"=w529:refnum<vi>, "error out"=w528:errorcluster)  [unwired: 5 out]
              n136 = Unbundle("Final Overvew Details") -> ("Size (m)"=w522:cluster{"Width":sgl, "Height":sgl}, "Pixels"=w521:i32, "Scan Speed (m/s)"=w516:sgl)
              n137 = call <userlib>:"Scan SetProperties.vi"("Application ref in"=w529, "Continuous scan"=enum16{"No change", "On", "Off"}."On", "Bouncy scan"=enum16{"No change", "On", "Off"}."On", "Error in (no error)"=w528) -> ("Application ref out"=w525:refnum<vi>, "Error out"=w524:errorcluster)  [unwired: 10 in]
              n138 = call <userlib>:"ScanBuffer Set.vi"("Application ref in"=w525, "Pixels"=w521, "error in (no error)"=w524) -> ("Application ref out"=w520:refnum<vi>, "error out"=w519:errorcluster)  [unwired: 11 in]
              n139 = Bundle("Scan Speed (m/s)"=w516, "Backward"=sgl nan) -> (w514:cluster{"Scan Speed (m/s)":sgl, "Backward":sgl})  [unwired: 1 in]
              n140 = call <userlib>:"ScanFrame Set.vi"("Application ref in"=w520, "Size (m)"=w522, "error in (no error)"=w519) -> ("Application ref out"=w518:refnum<vi>, "error out"=w517:errorcluster)  [unwired: 11 in]
              n141 = call <userlib>:"Speed Set.vi"("Application ref in"=w518, "Speed (m/s)"=w514, "error in (no error)"=w517) -> ("Application ref out"=w505:refnum<vi>, "error out"=w504:errorcluster)  [unwired: 11 in]
              n142 = call <userlib>:"Scan Action.vi"("error in (no error)"=w504, "Scan action (Start)"=enum16{"Start", "Stop", "Pause", "Resume"}."Start", "Application ref in"=w505) -> ("error out"=w501:errorcluster, "Application ref out"=w502:refnum<vi>)  [unwired: 6 in]
              n143 = Unbundle(w513) -> ("Corner Coords"=w512:cluster{"Corner x":sgl, "Corner y":sgl}, "Tip Shaping Position"=w511:cluster{"Tip x (m)":sgl, "Tip y (m)":sgl}, "Session path"=w510:path, "Filenames"=w509:cluster{"Filename 1":path, "Filename 2":path}, "Downscale Info"=w508:T6)  [unwired: 2 out]
              n144 = Bundle("Application ref out"=w502, "error out"=w501, "Corner Coords"=w512, "Tip Shaping Position"=w511, "Session path"=w510, "Filenames"=w509, "Downscale Info"=w508) -> (w507:T5)  [unwired: 1 in]
            }
          }
          "Vx vs. Scan #" <- w24
          "Vy vs. Scan #" <- w23
          "Shaping\nAttempts" <- w34
        }
      }
    }
  }
